vi "Testing Buffers.vi"() -> ()   [LabVIEW 2015]
uses:
  <instrlib>/_niInstr/DSP/v1/Shared/Public/IQ Data.ctl
  <instrlib>/_niInstr/Basic Elements/v1/FPGA/Private/Count Down U16.vi
  <instrlib>/_niInstr/Basic Elements/v1/FPGA/Private/Count Up U16.vi
  <instrlib>/_niInstr/Basic Elements/v1/FPGA/Private/Count Up U32.vi
  DDC_7976R_v1.lvlib
  <vilib>/Analysis/NI_AALBase.lvlib
  <instrlib>/_niInstr/Basic Elements/v1/FPGA/niInstr Basic Elements v1 FPGA.lvlib
  <instrlib>/_niInstr/DSP/v1/Shared/niInstr DSP v1 Shared.lvlib
panel:
  in  "data 3":T1
  in  "Test Case":T2(ring)
  out "Numeric Control 2":i32
  in  "data 2":T1
  out "ratio (16?)":dbl
  out "cntr.1SPC-IQ":u32
  out "cntr.16xU32":u32
  out "appended array":dbl[][](graph)
  out "double precision float":dbl
  out "*(type *) &x":fxp<+/-,18,1> format="%.18g"
  out "Numeric Control":u32
  in  "data":T1
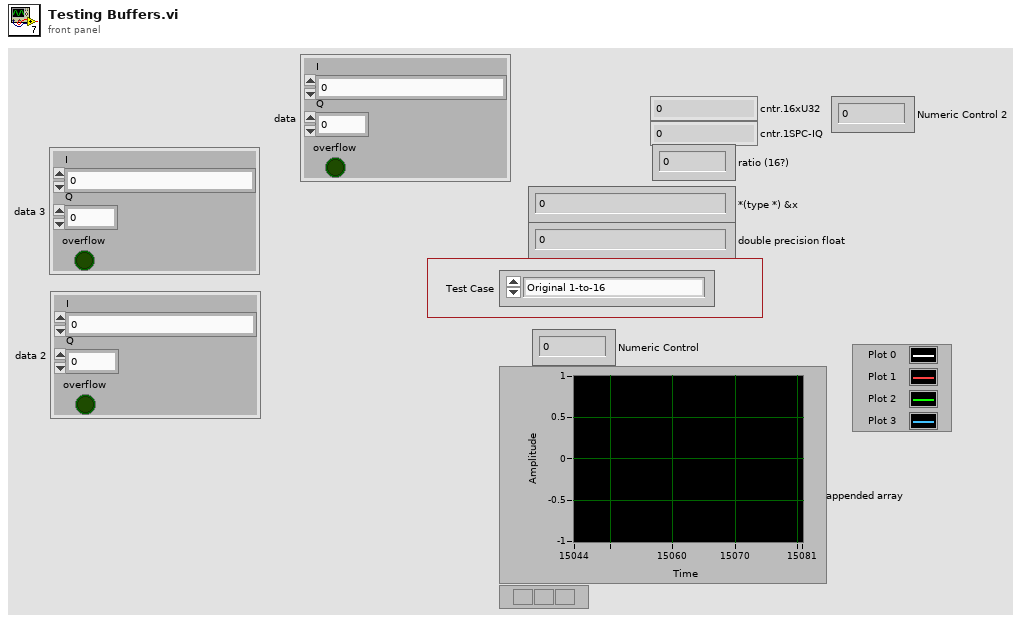
[diagram p1: front panel]
types:
  T1 = typedef "niInstr DSP v1 Shared.lvlib/IQ Data.ctl" = cluster{"I":fxp<+/-,18,1>, "Q":fxp<+/-,18,1>, "overflow":bool}
  T2 = enum16{"Original 1-to-16", "1ch", "2ch", "4ch", "8ch", "12ch", "16ch"}
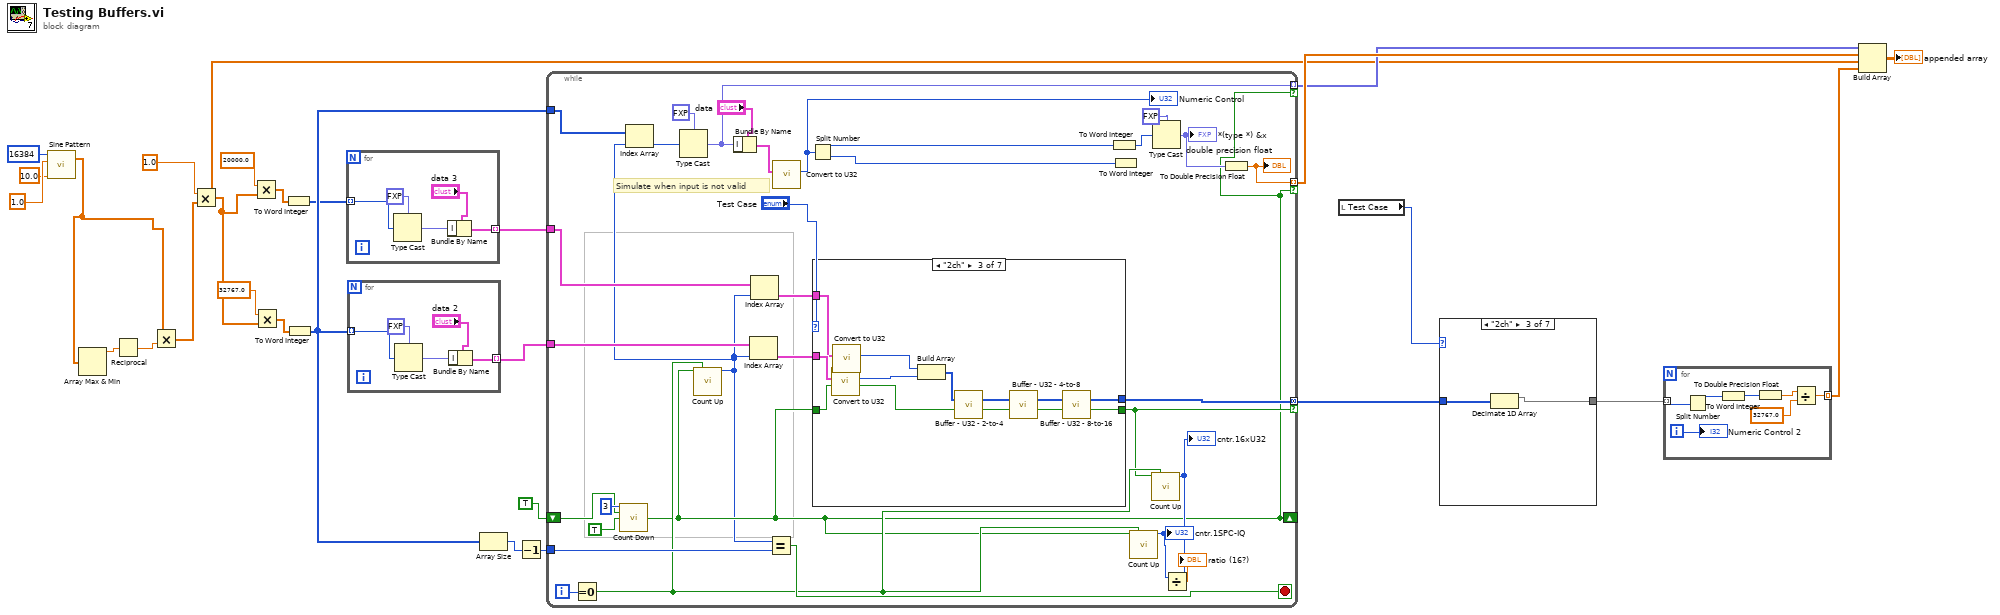
[diagram p0: block diagram]
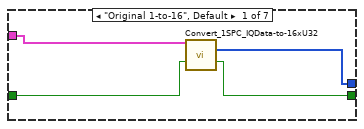
[diagram p8: hidden frame]
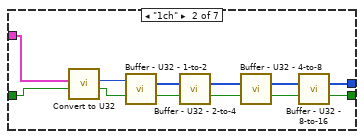
[diagram p9: hidden frame]
diagram:
  n1 = call <vilib>:"Sine Pattern.vi"("cycles"=10.0, "amplitude"=1.0 ("standard deviation"), "samples"=16384) -> ("Sinusoidal Pattern"=w20:dbl[])  [unwired: 1 in, 1 out]
  n2 = Array Max & Min(array=w20) -> (max value=w21:dbl)  [unwired: 3 out]
  n3 = Reciprocal(x=w21) -> (1/x=w19:dbl)
  n4 = Multiply(x=w20, y=w19) -> (x*y=w18:dbl[])
  n5 = Multiply(x=1.0, y=w18) -> (x*y=w2:dbl[])
  n6 = Multiply(x=20000.0, y=w2) -> (x*y=w4:dbl[])
  n7 = Multiply(x=32767.0, y=w2) -> (x*y=w16:dbl[])
  n8 = To Word Integer(number=w4) -> (16bit integer=w5:i16[])
  n9 = To Word Integer(number=w16) -> (16bit integer=w9:i16[])
  n10 = for {
    tunnel: w5 -> [w29] mode=indexing
    tunnel: [w28] -> w1 mode=indexing
    n11 = Type Cast(type=fxp<+/-,18,1> 0.0 ("I"), x=w29) -> (*(type *) &x=w32:fxp<+/-,18,1>)
    n12 = Bundle By Name(cluster="data 3", "I"=w32) -> (w28:T1)
  }
  n13 = for {
    tunnel: w9 -> [w34] mode=indexing
    tunnel: [w33] -> w10 mode=indexing
    n14 = Type Cast(type=fxp<+/-,18,1> 0.0 ("I"), x=w34) -> (*(type *) &x=w37:fxp<+/-,18,1>)
    n15 = Bundle By Name(cluster="data 2", "I"=w37) -> (w33:T1)
  }
  n16 = Array Size(array=w9) -> (size(s)=w12:i32)
  n17 = Decrement(x=w12) -> (x-1=w11:i32)
  n18 = while {
    tunnel: [w61] -> w26 mode=indexing if=w42
    tunnel: [w60] -> w24 mode=indexing if=w42
    tunnel: [w58] -> w8 mode=concatenating if=w44
    tunnel: w10 -> [w51]
    shift-right: [w42] -> _
    shift-left: TRUE -> [w50]
    tunnel: w11 -> [w48]
    tunnel: w9 -> [w46]
    tunnel: w1 -> [w40]
    i -> [w57]
    stop <- w49 stop-if-true
    # "Simulate when input is not valid"
    n19 = Equal To 0?(x=w57) -> (x = 0?=w47:bool)
    n20 = call-poly <instrlib>:"Count Down.vi"("count in"=u16 3, "load"=w50, "decrement"=TRUE) -> ("terminal count"=w42:bool)  [unwired: 11 in, 1 out]
    n21 = call-poly <instrlib>:"Count Up.vi"("increment"=w42, "reset"=w47) -> ("count out"=w39:u16)  [unwired: 13 in]
    n22 = Index Array(array=w46, index=w39) -> (element=w45:i16)
    n23 = Type Cast(type=fxp<+/-,18,1> 0.0 ("I"), x=w45) -> (*(type *) &x=w60:fxp<+/-,18,1>)
    n24 = Bundle By Name(cluster="data", "I"=w60) -> (w59:T1)
    n25 = Index Array(array=w51, index=w39) -> (element=w43:T1)
    n26 = Index Array(array=w40, index=w39) -> (element=w38:T1)
    n27 = Equal?(x=w39, y=w48) -> (x = y?=w49:bool)
    n28 = call "Convert to U32.vi"("IQData in"=w59) -> ("U32 out"=w69:u32)  [unwired: 8 in, 2 out]
    "Numeric Control" <- w69
    n29 = Split Number(x=w69) -> (hi(x)=w68:u16, lo(x)=w67:u16)
    n30 = case shown="\"2ch\"" "Test Case" {
      tunnel: [w70 w75 w91 _ _ _ _] -> w58
      tunnel: [w71 w74 w90 _ _ _ _] -> w44
      tunnel: w43 -> [w73 w85 w87 _ _ _ _]
      tunnel: w42 -> [w72 w84 w89 _ _ _ _]
      tunnel: w38 -> [_ _ w86 _ _ _ _]
      frame "Original 1-to-16", Default {
        n31 = call "Convert_1SPC_IQData-to-16xU32.vi"("1SPC-IQ in"=w73, "Input valid"=w72) -> ("16xU32"=w70:u32[], "Output valid"=w71:bool)  [unwired: 11 in, 1 out]
      }
      frame "1ch" {
        n32 = call "Convert to U32.vi"("input valid"=w84, "IQData in"=w85) -> ("output valid"=w79:bool, "U32 out"=w83:u32)  [unwired: 7 in, 1 out]
        n33 = call "Buffer - U32 - 1-to-2.vi"("U32 in"=w83, "Input valid"=w79) -> ("Array 2 out"=w82:u32[], "Output valid"=w78:bool)  [unwired: 12 in]
        n34 = call "Buffer - U32 - 2-to-4.vi"("Array 2 in"=w82, "Input valid"=w78) -> ("Array4 out"=w81:u32[], "Output valid"=w77:bool)  [unwired: 12 in]
        n35 = call "Buffer - U32 - 4-to-8.vi"("Array4in"=w81, "Input valid"=w77) -> ("Array8 out"=w80:u32[], "Output valid"=w76:bool)  [unwired: 12 in]
        n36 = call "Buffer - U32 - 8-to-16.vi"("Array 8 in"=w80, "Input valid"=w76) -> ("Array 16 out"=w75:u32[], "Output valid"=w74:bool)  [unwired: 12 in]
      }
      frame "2ch" {
        n37 = call "Convert to U32.vi"("input valid"=w89, "IQData in"=w87) -> ("output valid"=w92:bool, "U32 out"=w88:u32)  [unwired: 7 in, 1 out]
        n38 = call "Convert to U32.vi"("IQData in"=w86) -> ("U32 out"=w94:u32)  [unwired: 8 in, 2 out]
        n39 = Build Array(w94, w88) -> (w93:u32[])
        n40 = call "Buffer - U32 - 2-to-4.vi"("Array 2 in"=w93, "Input valid"=w92) -> ("Array4 out"=w98:u32[], "Output valid"=w96:bool)  [unwired: 12 in]
        n41 = call "Buffer - U32 - 4-to-8.vi"("Array4in"=w98, "Input valid"=w96) -> ("Array8 out"=w97:u32[], "Output valid"=w95:bool)  [unwired: 12 in]
        n42 = call "Buffer - U32 - 8-to-16.vi"("Array 8 in"=w97, "Input valid"=w95) -> ("Array 16 out"=w91:u32[], "Output valid"=w90:bool)  [unwired: 12 in]
      }
      frame "4ch" {
      }
      frame "8ch" {
      }
      frame "12ch" {
      }
      frame "16ch" {
      }
    }
    n43 = To Word Integer(number=w68) -> (16bit integer=w66:i16)
    n44 = To Word Integer(number=w67) -> ()  [unwired: 1 out]
    n45 = call-poly <instrlib>:"Count Up.vi"("increment"=w42, "reset"=w47) -> ("count out"=w56:u32)  [unwired: 13 in]
    "cntr.1SPC-IQ" <- w56
    n46 = call-poly <instrlib>:"Count Up.vi"("increment"=w44, "reset"=w47) -> ("count out"=w55:u32)  [unwired: 13 in]
    "cntr.16xU32" <- w55
    n47 = Type Cast(type=fxp<+/-,18,1> 0.0 ("I"), x=w66) -> (*(type *) &x=w64:fxp<+/-,18,1>)
    "*(type *) &x" <- w64
    n48 = Divide(x=w56, y=w55) -> (x/y=→"ratio (16?)":dbl)
    n49 = To Double Precision Float(number=w64) -> (double precision float=w61:dbl)
    "double precision float" <- w61
  }
  n50 = local read "Test Case"() -> (w6:T2)
  n51 = case shown="\"2ch\"" w6 {
    tunnel: w8 -> [w99 w100 w102 w103 w104 w105 w106]
    tunnel: [w99 w100 w101 w103 w104 w105 w106] -> w7
    frame "Original 1-to-16", Default {
    }
    frame "1ch" {
    }
    frame "2ch" {
      n52 = Decimate 1D Array(w102) -> (w101:u32[])  [unwired: 1 out]
    }
    frame "4ch" {
    }
    frame "8ch" {
    }
    frame "12ch" {
    }
    frame "16ch" {
    }
  }
  n53 = for {
    tunnel: w7 -> [w113] mode=indexing
    tunnel: [w108] -> w14 mode=indexing
    i -> [w107]
    n54 = Split Number(x=w113) -> (hi(x)=w112:u16)  [unwired: 1 out]
    n55 = To Word Integer(number=w112) -> (16bit integer=w109:i16)
    n56 = To Double Precision Float(number=w109) -> (double precision float=w111:dbl)
    n57 = Divide(x=w111, y=32767.0) -> (x/y=w108:dbl)
    "Numeric Control 2" <- w107
  }
  n58 = Build Array(w24, w26, w2, w14) -> (→"appended array":dbl[][])
